vi "UTF string (SubVI).vi"(8 "error in":errorcluster, 11 "StringIn":string) -> (0 "error out":errorcluster, 3 "StringOut":string)   [LabVIEW 2017, in "LV_Unicorn.lvlib"]
uses:
  LV_Unicorn.lvlib
  <vilib>/addons/Tools/Unicode/UTF8 Tools.lvlib
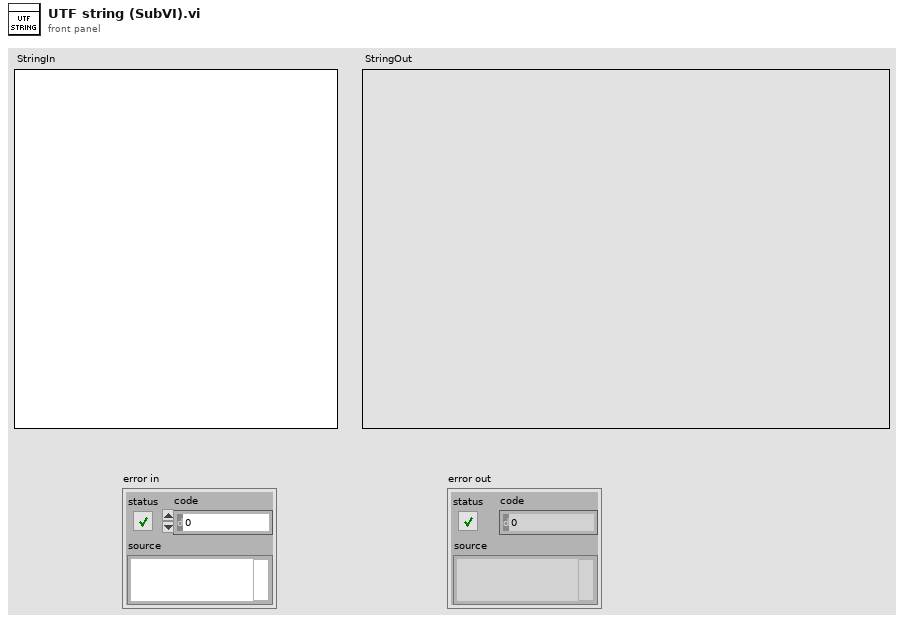
[diagram p1: front panel]
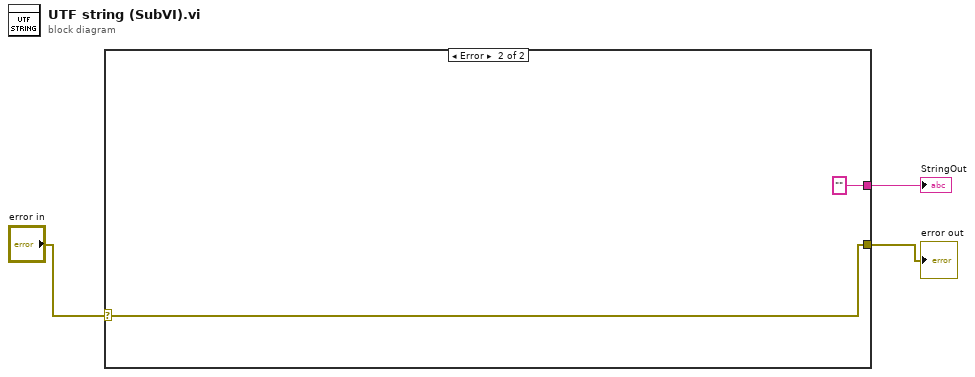
[diagram p0: block diagram]
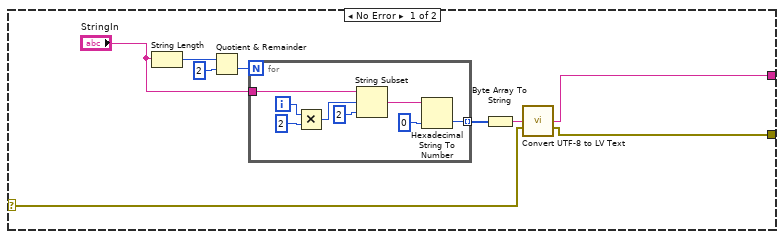
[diagram p2: hidden frame]
diagram:
  n1 = case shown="Error" "error in" {
    selector: "error in" -> [w6 w22]
    tunnel: [w5 w22] -> w2
    tunnel: [w4 "" ("LV Text")] -> w1
    frame No Error {
      n2 = String Length(string="StringIn") -> (length=w12:i32)
      n3 = Quotient & Remainder(x=w12, y=2) -> (floor(x/y)=w10:i32)  [unwired: 1 out]
      n4 = for {
        N: w10 -> [_]
        tunnel: [w20] -> w9 mode=indexing
        tunnel: "StringIn" -> [w15]
        i -> [w17]
        n5 = Multiply(x=w17, y=2) -> (x*y=w16:i32)
        n6 = String Subset(string=w15, offset (0)=w16, length (rest)=2 ("length (rest)")) -> (substring=w13:string)
        n7 = Hexadecimal String To Number(string=w13, default (0uL)=u8 0 ("default (0 U32)")) -> (number=w20:u8)  [unwired: 1 in, 1 out]
      }
      n8 = Byte Array To String(unsigned byte array=w9) -> (string=w7:string)
      n9 = call <vilib>:"Convert UTF-8 to LV Text.vi"("UTF-8 Text"=w7, "error in"=w6) -> ("LV Text"=w4:string, "error out"=w5:errorcluster)  [unwired: 12 in]
    }
    frame Error {
    }
  }
  "error out" <- w2
  "StringOut" <- w1
